vi "get_grating_info.vi"(4 "error in (no error)":errorcluster, 6 "grating name":string, 7 "configuration file path":path) -> (0 "error out":errorcluster, 2 "Grating Info":T1 {"thickness (mm)" format="%.2f"; "modulation" format="%.2f"})   [LabVIEW 2015]
uses:
  <vilib>/Utility/config.llb/Read Key (String).vi
  <vilib>/Utility/config.llb/Read Key (I32).vi
  <vilib>/Utility/config.llb/Read Key (Double).vi
  <vilib>/Utility/config.llb/NI_LVConfig.lvlib
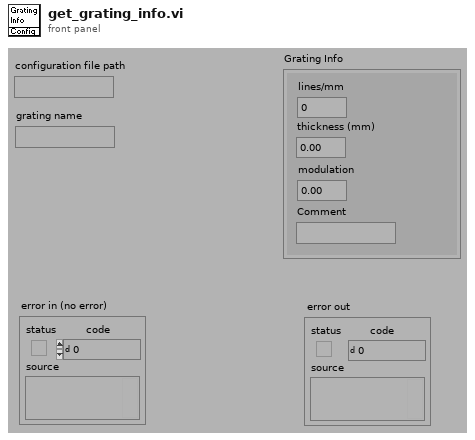
[diagram p1: front panel]
types:
  T1 = cluster{"Comment":string, "lines/mm":i32, "modulation":dbl, "thickness (mm)":dbl}
  T2 = typedef "NI_LVConfig.lvlib/Config Data RefNum.ctl" = refnum<k1>
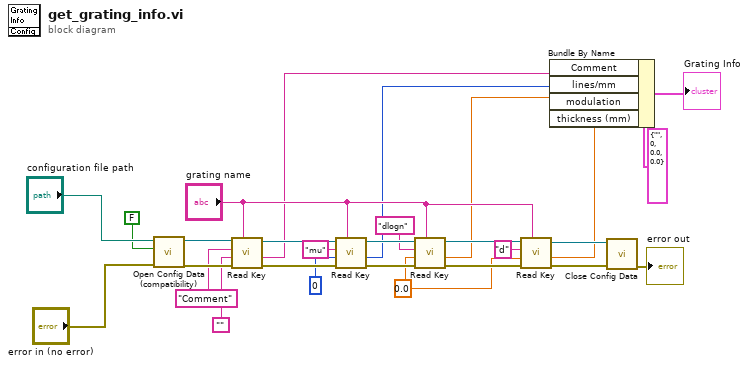
[diagram p0: block diagram]
diagram:
  w9 = 0.0
  n1 = call <vilib>:"Open Config Data (compatibility).vi"("error in (no error)"="error in (no error)", "create file if necessary (T)"=FALSE, "configuration file path"="configuration file path") -> ("error out"=w28:errorcluster, "refnum"=w27:T2)  [unwired: 6 in, 1 out]
  n2 = call-poly <vilib>:"Read Key.vi"("section"="grating name", "error in (no error)"=w28, "default value"="", "key"="Comment", "refnum"=w27) -> ("error out"=w20:errorcluster, "value"=w4:string, "refnum out"=w19:T2)  [unwired: 3 in, 1 out]
  n3 = call-poly <vilib>:"Read Key.vi"("section"="grating name", "error in (no error)"=w20, "default value"=0, "key"="mu", "refnum"=w19) -> ("error out"=w15:errorcluster, "value"=w3:i32, "refnum out"=w16:T2)  [unwired: 3 in, 1 out]
  n4 = call-poly <vilib>:"Read Key.vi"("section"="grating name", "error in (no error)"=w15, "default value"=w9, "key"="dlogn", "refnum"=w16) -> ("error out"=w12:errorcluster, "value"=w2:dbl, "refnum out"=w13:T2)  [unwired: 3 in, 1 out]
  n5 = call-poly <vilib>:"Read Key.vi"("section"="grating name", "error in (no error)"=w12, "default value"=w9, "key"="d", "refnum"=w13) -> ("error out"=w8:errorcluster, "value"=w1:dbl, "refnum out"=w7:T2)  [unwired: 3 in, 1 out]
  n6 = Bundle By Name(cluster=T1 {"Comment"="", "lines/mm"=0, "modulation"=0.0, "thickness (mm)"=0.0} ("Grating Info"), "Comment"=w4, "lines/mm"=w3, "modulation"=w2, "thickness (mm)"=w1) -> (→"Grating Info":T1)
  n7 = call <vilib>:"Close Config Data.vi"("error in (no error)"=w8, "refnum"=w7) -> ("error out"=→"error out":errorcluster)  [unwired: 8 in, 1 out]
